vi "Write User Info.vi"(8 "error in (no error)":errorcluster, 10 "User Info":T1, 11 "MQTT Client in":refnum<class "MQTT Client.lvclass">) -> (0 "error out":errorcluster, 3 "MQTT Client out":refnum<class "MQTT Client.lvclass">)   [LabVIEW 2020, in "MQTT Client.lvclass"]
uses:
  MQTT Client.lvclass
  mqttTypedef/UserCredentials.ctl
  MQTT Client.lvclass/MQTT Client.ctl
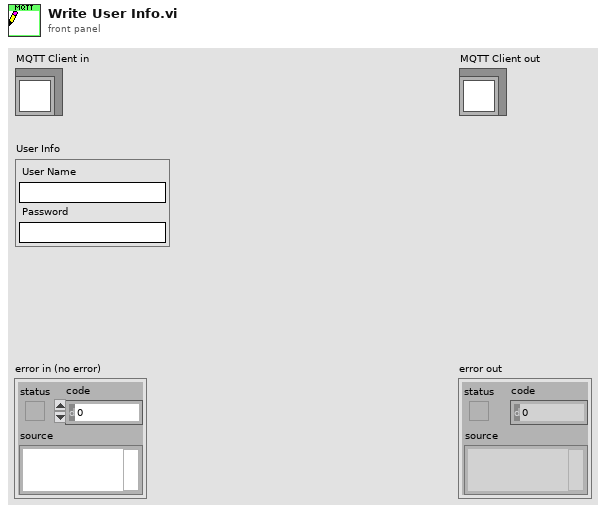
[diagram p1: front panel]
types:
  T1 = typedef "MQTT Client.lvclass/UserCredentials.ctl" = cluster{"User Name":string, "Password":string}
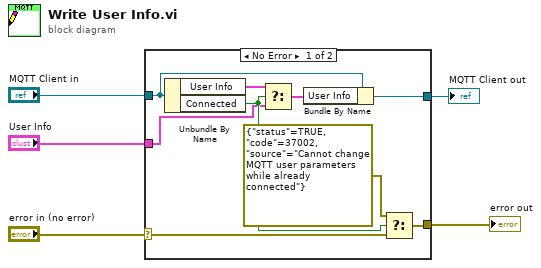
[diagram p0: block diagram]
diagram:
  n1 = case shown="No Error" "error in (no error)" {
    selector: "error in (no error)" -> [w12 w15]
    tunnel: [w11 w15] -> w1
    tunnel: [w14 w16] -> w4
    tunnel: "MQTT Client in" -> [w13 w16]
    tunnel: "User Info" -> [w7 _]
    frame No Error {
      n2 = Unbundle By Name(w13) -> ("User Info"=w9:T1, "Connected"=w8:bool)
      n3 = Select(t=w9, s=w8, f=w7) -> (s? t:f=w6:T1)
      n4 = Bundle By Name(cluster=w13, "User Info"=w6) -> (w14:refnum<class "MQTT Client.lvclass">)
      n5 = Select(t=errorcluster {"status"=TRUE, "code"=37002, "source"="Cannot change MQTT user parameters while already connected"}, s=w8, f=w12) -> (s? t:f=w11:errorcluster)
    }
    frame Error {
    }
  }
  "error out" <- w1
  "MQTT Client out" <- w4
